vi "LVCAM Msg Receive.vi"(11 "Self Actor in":refnum<class "Self Actor.lvclass">) -> (0 "error out":errorcluster, 1 "DeQ Msg?":bool, 2 "Msg":refnum<class "Msg.lvclass">, 3 "Self Actor out":refnum<class "Self Actor.lvclass">)   [LabVIEW 2021, in "LVCAM.lvlib" / "Self Actor.lvclass"]
uses:
  Self Actor.lvclass
  Msg/Msg.lvclass
  Self Actor.lvclass/Self Actor.ctl
  Msgs/LVCAM Nest Destroyed/LVCAM Nest Destroyed Msg/LVCAM Nest Destroyed Msg.lvclass
  C:/PPLs/LabVIEW-Composed-Actor-Model-LVCAM/LabVIEW-Composed-Actor-Model-LVCAM/LVCAM/LVCAM/Msg/Msg.lvclass
  Msgs/LVCAM Destroy Self/LVCAM Destroy Self Msg/LVCAM Destroy Self Msg.lvclass
  Msg Q/Msg Q.lvclass
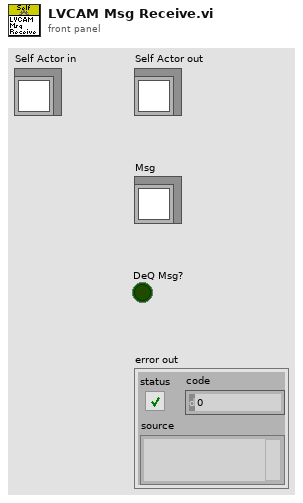
[diagram p1: front panel]
types:
  T1 = typedef "LVCAM.lvlib/Self Actor.lvclass/State.ctl" = enum16{"Safe Msging", "Destroying Self"}
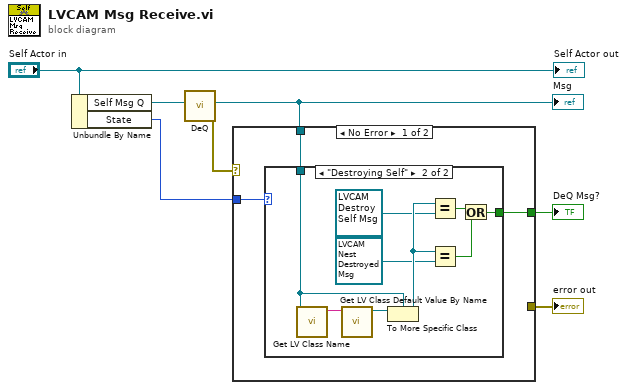
[diagram p0: block diagram]
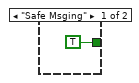
[diagram p2: hidden frame]
diagram:
  n1 = Unbundle By Name("Self Actor in") -> ("Self Msg Q"=w2:refnum<data-value>, "State"=w6:T1)
  n2 = call "DeQ.vi"("Msg Q"=w2) -> ("error out"=w1:errorcluster, "Msg"=w3:refnum<class "Msg.lvclass">)  [unwired: 9 in]
  "Msg" <- w3
  n3 = case shown="No Error" w1 {
    selector: w1 -> [_ w21]
    tunnel: w3 -> [w8 _]
    tunnel: [w9 _] -> w7
    tunnel: w6 -> [w10 _]
    tunnel: [_ w21] -> w5
    frame No Error {
      n4 = case shown="\"Destroying Self\"" w10 {
        tunnel: w8 -> [_ w17]
        tunnel: [TRUE w14] -> w9
        frame "Safe Msging" {
        }
        frame "Destroying Self" {
          n5 = call <vilib>:"Get LV Class Name.vi"("object"=w17) -> ("class name"=w20:string)  [unwired: 9 in, 1 out]
          n6 = call <vilib>:"Get LV Class Default Value By Name.vi"("class name"=w20) -> ("object"=w19:refnum<class>)  [unwired: 9 in, 1 out]
          n7 = To More Specific Class(target class=w17, reference=w19) -> (specific class reference=w16:refnum<class "Msg.lvclass">)  [unwired: 1 in, 1 out]
          n8 = Equal?(x=w16, y=refnum<class "LVCAM Destroy Self Msg.lvclass"> refnum ("LVCAM Destroy Self.lvlib:LVCAM Destroy Self Msg.lvclass")) -> (x = y?=w18:bool)
          n9 = Equal?(x=w16, y=refnum<class "LVCAM Nest Destroyed Msg.lvclass"> refnum ("LVCAM Nest Destroyed.lvlib:LVCAM Nest Destroyed Msg.lvclass")) -> (x = y?=w13:bool)
          n10 = Or(x=w18, y=w13) -> (x .or. y?=w14:bool)
        }
      }
    }
    frame Error {
      # "#LVCAM Error"
    }
  }
  "DeQ Msg?" <- w7
  "error out" <- w5
  "Self Actor out" <- "Self Actor in"
